vi "Lab Panel V4.82.vi"() -> ()   [LabVIEW 2013] (continued)
                            n1335 = Bundle(cluster=w2277) -> (w2276:T4)  [unwired: 3 in]
                            n1336 = local write "DISP LAB01-1"(w2276) -> ()
                            n1337 = local write "O/I  LAB01-1"(w2274) -> ()
                            n1338 = local write "run lab01-1"(w2274) -> ()
                            n1339 = local write "RUN LAB01-1"(w2274) -> ()
                          }
                          frame #1 {
                            n1340 = TDMS Close(11:w2279) -> (0:w2278:errorcluster)  [unwired: 1 in, 1 out]
                            n1341 = local write "data file error"(w2278) -> ()
                          }
                          frame #2 {
                            n1342 = stacked-sequence {
                              tunnel: "LAB01-1" -> [w2282 w2284]
                              frame #0 {
                                n1343 = call "sub vi - defrag tdms v1.vi"("panel id"=w2282) -> ("error out"=w2281:errorcluster)  [unwired: 10 in]
                                n1344 = local write "data file error"(w2281) -> ()
                              }
                              frame #1 {
                                n1345 = call "Save data file to network drive v1.vi"("panel id"=w2284) -> ("network file save error"=w2283:errorcluster)  [unwired: 9 in, 1 out]
                                n1346 = local write "data file error"(w2283) -> ()
                              }
                            }
                          }
                        }
                      }
                    }
                  }
                }
              }
              frame #1 {
                # "LAB01-2"
                n1347 = local read "run lab01-2"() -> (w2285:bool)
                n1348 = case shown="True" w2285 {
                  frame False {
                  }
                  frame True {
                    n1349 = local read "DISP LAB01-2"() -> (w2292:T4)
                    n1350 = local read "TDMS LAB01-2"() -> (w2291:refnum<k34>)
                    n1351 = Unbundle(w2292) -> ("CYCLE"=w2288:dbl, "STATUS"=w2293:string)  [unwired: 1 out]
                    n1352 = Not Equal?(x=w2293, y="RUN") -> (x != y?=w2287:bool)
                    n1353 = Greater?(x=w2288, y=2.0) -> (0:w2289:bool)
                    n1354 = And(x=w2289, y=w2287) -> (x .and. y?=w2286:bool)
                    n1355 = case shown="True" w2286 {
                      tunnel: w2292 -> [_ w2296]
                      tunnel: w2291 -> [_ w2295]
                      frame False {
                      }
                      frame True {
                        n1356 = stacked-sequence {
                          tunnel: w2296 -> [w2299 _ _]
                          tunnel: w2295 -> [_ w2301 _]
                          frame #0 {
                            w2297 = FALSE
                            n1357 = local write "mail control"("END") -> ()
                            n1358 = Bundle(cluster=w2299) -> (w2300:T4)  [unwired: 3 in]
                            n1359 = local write "RUN LAB01-2"(w2297) -> ()
                            n1360 = local write "run lab01-2"(w2297) -> ()
                            n1361 = local write "O/I  LAB01-2"(w2297) -> ()
                            n1362 = local write "DISP LAB01-2"(w2300) -> ()
                          }
                          frame #1 {
                            n1363 = TDMS Close(11:w2301) -> (0:w2302:errorcluster)  [unwired: 1 in, 1 out]
                            n1364 = local write "data file error"(w2302) -> ()
                          }
                          frame #2 {
                            n1365 = stacked-sequence {
                              tunnel: "LAB01-2" -> [w2305 w2307]
                              frame #0 {
                                n1366 = call "sub vi - defrag tdms v1.vi"("panel id"=w2305) -> ("error out"=w2304:errorcluster)  [unwired: 10 in]
                                n1367 = local write "data file error"(w2304) -> ()
                              }
                              frame #1 {
                                n1368 = call "Save data file to network drive v1.vi"("panel id"=w2307) -> ("network file save error"=w2306:errorcluster)  [unwired: 9 in, 1 out]
                                n1369 = local write "data file error"(w2306) -> ()
                              }
                            }
                          }
                        }
                      }
                    }
                  }
                }
              }
              frame #2 {
                # "LAB02-1"
                n1370 = local read "run lab02-1"() -> (w2308:bool)
                n1371 = case shown="True" w2308 {
                  frame False {
                  }
                  frame True {
                    n1372 = local read "DISP LAB02-1"() -> (w2315:T4)
                    n1373 = Unbundle(w2315) -> ("CYCLE"=w2311:dbl, "STATUS"=w2316:string)  [unwired: 1 out]
                    n1374 = local read "TDMS LAB02-1"() -> (w2314:refnum<k34>)
                    n1375 = Not Equal?(x=w2316, y="RUN") -> (x != y?=w2310:bool)
                    n1376 = Greater?(x=w2311, y=2.0) -> (0:w2312:bool)
                    n1377 = And(x=w2312, y=w2310) -> (x .and. y?=w2309:bool)
                    n1378 = case shown="True" w2309 {
                      tunnel: w2315 -> [_ w2319]
                      tunnel: w2314 -> [_ w2318]
                      frame False {
                      }
                      frame True {
                        n1379 = stacked-sequence {
                          tunnel: w2319 -> [w2322 _ _]
                          tunnel: w2318 -> [_ w2324 _]
                          frame #0 {
                            w2320 = FALSE
                            n1380 = local write "mail control"("END") -> ()
                            n1381 = Bundle(cluster=w2322) -> (w2323:T4)  [unwired: 3 in]
                            n1382 = local write "O/I  LAB02-1"(w2320) -> ()
                            n1383 = local write "RUN LAB02-1"(w2320) -> ()
                            n1384 = local write "run lab02-1"(w2320) -> ()
                            n1385 = local write "DISP LAB02-1"(w2323) -> ()
                          }
                          frame #1 {
                            n1386 = TDMS Close(11:w2324) -> (0:w2325:errorcluster)  [unwired: 1 in, 1 out]
                            n1387 = local write "data file error"(w2325) -> ()
                          }
                          frame #2 {
                            n1388 = stacked-sequence {
                              tunnel: "LAB02-1" -> [w2328 w2330]
                              frame #0 {
                                n1389 = call "sub vi - defrag tdms v1.vi"("panel id"=w2328) -> ("error out"=w2327:errorcluster)  [unwired: 10 in]
                                n1390 = local write "data file error"(w2327) -> ()
                              }
                              frame #1 {
                                n1391 = call "Save data file to network drive v1.vi"("panel id"=w2330) -> ("network file save error"=w2329:errorcluster)  [unwired: 9 in, 1 out]
                                n1392 = local write "data file error"(w2329) -> ()
                              }
                            }
                          }
                        }
                      }
                    }
                  }
                }
              }
              frame #3 {
                # "LAB02-2"
                n1393 = local read "run lab02-2"() -> (w2331:bool)
                n1394 = case shown="True" w2331 {
                  frame False {
                  }
                  frame True {
                    n1395 = local read "DISP LAB02-2"() -> (w2338:T4)
                    n1396 = local read "TDMS LAB02-2"() -> (w2337:refnum<k34>)
                    n1397 = Unbundle(w2338) -> ("CYCLE"=w2334:dbl, "STATUS"=w2339:string)  [unwired: 1 out]
                    n1398 = Not Equal?(x=w2339, y="RUN") -> (x != y?=w2333:bool)
                    n1399 = Greater?(x=w2334, y=2.0) -> (0:w2335:bool)
                    n1400 = And(x=w2335, y=w2333) -> (x .and. y?=w2332:bool)
                    n1401 = case shown="True" w2332 {
                      tunnel: w2338 -> [_ w2342]
                      tunnel: w2337 -> [_ w2341]
                      frame False {
                      }
                      frame True {
                        n1402 = stacked-sequence {
                          tunnel: w2342 -> [w2345 _ _]
                          tunnel: w2341 -> [_ w2347 _]
                          frame #0 {
                            w2343 = FALSE
                            n1403 = local write "mail control"("END") -> ()
                            n1404 = Bundle(cluster=w2345) -> (w2346:T4)  [unwired: 3 in]
                            n1405 = local write "O/I  LAB02-2"(w2343) -> ()
                            n1406 = local write "run lab02-2"(w2343) -> ()
                            n1407 = local write "RUN LAB02-2"(w2343) -> ()
                            n1408 = local write "DISP LAB02-2"(w2346) -> ()
                          }
                          frame #1 {
                            n1409 = TDMS Close(11:w2347) -> (0:w2348:errorcluster)  [unwired: 1 in, 1 out]
                            n1410 = local write "data file error"(w2348) -> ()
                          }
                          frame #2 {
                            n1411 = stacked-sequence {
                              tunnel: "LAB02-2" -> [w2351 w2353]
                              frame #0 {
                                n1412 = call "sub vi - defrag tdms v1.vi"("panel id"=w2351) -> ("error out"=w2350:errorcluster)  [unwired: 10 in]
                                n1413 = local write "data file error"(w2350) -> ()
                              }
                              frame #1 {
                                n1414 = call "Save data file to network drive v1.vi"("panel id"=w2353) -> ("network file save error"=w2352:errorcluster)  [unwired: 9 in, 1 out]
                                n1415 = local write "data file error"(w2352) -> ()
                              }
                            }
                          }
                        }
                      }
                    }
                  }
                }
              }
              frame #4 {
                # "LAB03-1"
                n1416 = local read "run lab03-1"() -> (w2354:bool)
                n1417 = case shown="True" w2354 {
                  frame False {
                  }
                  frame True {
                    n1418 = local read "DISP LAB03-1"() -> (w2361:T4)
                    n1419 = local read "TDMS LAB03-1"() -> (w2360:refnum<k34>)
                    n1420 = Unbundle(w2361) -> ("CYCLE"=w2357:dbl, "STATUS"=w2362:string)  [unwired: 1 out]
                    n1421 = Not Equal?(x=w2362, y="RUN") -> (x != y?=w2356:bool)
                    n1422 = Greater?(x=w2357, y=2.0) -> (0:w2358:bool)
                    n1423 = And(x=w2358, y=w2356) -> (x .and. y?=w2355:bool)
                    n1424 = case shown="True" w2355 {
                      tunnel: w2361 -> [_ w2365]
                      tunnel: w2360 -> [_ w2364]
                      frame False {
                      }
                      frame True {
                        n1425 = stacked-sequence {
                          tunnel: w2365 -> [w2368 _ _]
                          tunnel: w2364 -> [_ w2370 _]
                          frame #0 {
                            w2366 = FALSE
                            n1426 = local write "mail control"("END") -> ()
                            n1427 = Bundle(cluster=w2368) -> (w2369:T4)  [unwired: 3 in]
                            n1428 = local write "O/I  LAB03-1"(w2366) -> ()
                            n1429 = local write "run lab03-1"(w2366) -> ()
                            n1430 = local write "RUN LAB03-1"(w2366) -> ()
                            n1431 = local write "DISP LAB03-1"(w2369) -> ()
                          }
                          frame #1 {
                            n1432 = TDMS Close(11:w2370) -> (0:w2371:errorcluster)  [unwired: 1 in, 1 out]
                            n1433 = local write "data file error"(w2371) -> ()
                          }
                          frame #2 {
                            n1434 = stacked-sequence {
                              tunnel: "LAB03-1" -> [w2374 w2376]
                              frame #0 {
                                n1435 = call "sub vi - defrag tdms v1.vi"("panel id"=w2374) -> ("error out"=w2373:errorcluster)  [unwired: 10 in]
                                n1436 = local write "data file error"(w2373) -> ()
                              }
                              frame #1 {
                                n1437 = call "Save data file to network drive v1.vi"("panel id"=w2376) -> ("network file save error"=w2375:errorcluster)  [unwired: 9 in, 1 out]
                                n1438 = local write "data file error"(w2375) -> ()
                              }
                            }
                          }
                        }
                      }
                    }
                  }
                }
              }
              frame #5 {
                # "LAB03-2"
                n1439 = local read "run lab03-2"() -> (w2377:bool)
                n1440 = case shown="True" w2377 {
                  frame False {
                  }
                  frame True {
                    n1441 = local read "DISP LAB03-2"() -> (w2384:T4)
                    n1442 = Unbundle(w2384) -> ("CYCLE"=w2380:dbl, "STATUS"=w2385:string)  [unwired: 1 out]
                    n1443 = local read "TDMS LAB03-2"() -> (w2383:refnum<k34>)
                    n1444 = Not Equal?(x=w2385, y="RUN") -> (x != y?=w2379:bool)
                    n1445 = Greater?(x=w2380, y=2.0) -> (0:w2381:bool)
                    n1446 = And(x=w2381, y=w2379) -> (x .and. y?=w2378:bool)
                    n1447 = case shown="True" w2378 {
                      tunnel: w2384 -> [_ w2388]
                      tunnel: w2383 -> [_ w2387]
                      frame False {
                      }
                      frame True {
                        n1448 = stacked-sequence {
                          tunnel: w2388 -> [w2391 _ _]
                          tunnel: w2387 -> [_ w2393 _]
                          frame #0 {
                            w2389 = FALSE
                            n1449 = local write "mail control"("END") -> ()
                            n1450 = Bundle(cluster=w2391) -> (w2392:T4)  [unwired: 3 in]
                            n1451 = local write "RUN LAB03-2"(w2389) -> ()
                            n1452 = local write "O/I  LAB03-2"(w2389) -> ()
                            n1453 = local write "DISP LAB03-2"(w2392) -> ()
                            n1454 = local write "run lab03-2"(w2389) -> ()
                          }
                          frame #1 {
                            n1455 = TDMS Close(11:w2393) -> (0:w2394:errorcluster)  [unwired: 1 in, 1 out]
                            n1456 = local write "data file error"(w2394) -> ()
                          }
                          frame #2 {
                            n1457 = stacked-sequence {
                              tunnel: "LAB03-2" -> [w2397 w2399]
                              frame #0 {
                                n1458 = call "sub vi - defrag tdms v1.vi"("panel id"=w2397) -> ("error out"=w2396:errorcluster)  [unwired: 10 in]
                                n1459 = local write "data file error"(w2396) -> ()
                              }
                              frame #1 {
                                n1460 = call "Save data file to network drive v1.vi"("panel id"=w2399) -> ("network file save error"=w2398:errorcluster)  [unwired: 9 in, 1 out]
                                n1461 = local write "data file error"(w2398) -> ()
                              }
                            }
                          }
                        }
                      }
                    }
                  }
                }
              }
              frame #6 {
                # "LAB04-1"
                n1462 = local read "run lab04-1"() -> (w2400:bool)
                n1463 = case shown="True" w2400 {
                  frame False {
                  }
                  frame True {
                    n1464 = local read "DISP LAB04-1"() -> (w2407:T4)
                    n1465 = Unbundle(w2407) -> ("CYCLE"=w2403:dbl, "STATUS"=w2408:string)  [unwired: 1 out]
                    n1466 = local read "TDMS LAB04-1"() -> (w2406:refnum<k34>)
                    n1467 = Not Equal?(x=w2408, y="RUN") -> (x != y?=w2402:bool)
                    n1468 = Greater?(x=w2403, y=2.0) -> (0:w2404:bool)
                    n1469 = And(x=w2404, y=w2402) -> (x .and. y?=w2401:bool)
                    n1470 = case shown="True" w2401 {
                      tunnel: w2407 -> [_ w2411]
                      tunnel: w2406 -> [_ w2410]
                      frame False {
                      }
                      frame True {
                        n1471 = stacked-sequence {
                          tunnel: w2411 -> [w2414 _ _]
                          tunnel: w2410 -> [_ w2416 _]
                          frame #0 {
                            w2412 = FALSE
                            n1472 = local write "mail control"("END") -> ()
                            n1473 = Bundle(cluster=w2414) -> (w2415:T4)  [unwired: 3 in]
                            n1474 = local write "RUN LAB04-1"(w2412) -> ()
                            n1475 = local write "O/I  LAB04-1"(w2412) -> ()
                            n1476 = local write "run lab04-1"(w2412) -> ()
                            n1477 = local write "DISP LAB04-1"(w2415) -> ()
                          }
                          frame #1 {
                            n1478 = TDMS Close(11:w2416) -> (0:w2417:errorcluster)  [unwired: 1 in, 1 out]
                            n1479 = local write "data file error"(w2417) -> ()
                          }
                          frame #2 {
                            n1480 = stacked-sequence {
                              tunnel: "LAB04-1" -> [w2420 w2422]
                              frame #0 {
                                n1481 = call "sub vi - defrag tdms v1.vi"("panel id"=w2420) -> ("error out"=w2419:errorcluster)  [unwired: 10 in]
                                n1482 = local write "data file error"(w2419) -> ()
                              }
                              frame #1 {
                                n1483 = call "Save data file to network drive v1.vi"("panel id"=w2422) -> ("network file save error"=w2421:errorcluster)  [unwired: 9 in, 1 out]
                                n1484 = local write "data file error"(w2421) -> ()
                              }
                            }
                          }
                        }
                      }
                    }
                  }
                }
              }
              frame #7 {
                # "LAB04-2"
                n1485 = local read "run lab04-2"() -> (w2423:bool)
                n1486 = case shown="True" w2423 {
                  frame False {
                  }
                  frame True {
                    n1487 = local read "DISP LAB04-2"() -> (w2430:T4)
                    n1488 = Unbundle(w2430) -> ("CYCLE"=w2426:dbl, "STATUS"=w2431:string)  [unwired: 1 out]
                    n1489 = Not Equal?(x=w2431, y="RUN") -> (x != y?=w2425:bool)
                    n1490 = local read "TDMS LAB04-2"() -> (w2429:refnum<k34>)
                    n1491 = Greater?(x=w2426, y=2.0) -> (0:w2427:bool)
                    n1492 = And(x=w2427, y=w2425) -> (x .and. y?=w2424:bool)
                    n1493 = case shown="True" w2424 {
                      tunnel: w2430 -> [_ w2434]
                      tunnel: w2429 -> [_ w2433]
                      frame False {
                      }
                      frame True {
                        n1494 = stacked-sequence {
                          tunnel: w2434 -> [w2437 _ _]
                          tunnel: w2433 -> [_ w2439 _]
                          frame #0 {
                            w2435 = FALSE
                            n1495 = local write "mail control"("END") -> ()
                            n1496 = Bundle(cluster=w2437) -> (w2438:T4)  [unwired: 3 in]
                            n1497 = local write "O/I  LAB04-2"(w2435) -> ()
                            n1498 = local write "RUN LAB04-2"(w2435) -> ()
                            n1499 = local write "run lab04-2"(w2435) -> ()
                            n1500 = local write "DISP LAB04-2"(w2438) -> ()
                          }
                          frame #1 {
                            n1501 = TDMS Close(11:w2439) -> (0:w2440:errorcluster)  [unwired: 1 in, 1 out]
                            n1502 = local write "data file error"(w2440) -> ()
                          }
                          frame #2 {
                            n1503 = stacked-sequence {
                              tunnel: "LAB04-2" -> [w2443 w2445]
                              frame #0 {
                                n1504 = call "sub vi - defrag tdms v1.vi"("panel id"=w2443) -> ("error out"=w2442:errorcluster)  [unwired: 10 in]
                                n1505 = local write "data file error"(w2442) -> ()
                              }
                              frame #1 {
                                n1506 = call "Save data file to network drive v1.vi"("panel id"=w2445) -> ("network file save error"=w2444:errorcluster)  [unwired: 9 in, 1 out]
                                n1507 = local write "data file error"(w2444) -> ()
                              }
                            }
                          }
                        }
                      }
                    }
                  }
                }
              }
              frame #8 {
                # "LAB05-1"
                n1508 = local read "run lab05-1"() -> (w2446:bool)
                n1509 = case shown="True" w2446 {
                  frame False {
                  }
                  frame True {
                    n1510 = local read "DISP LAB05-1"() -> (w2453:T4)
                    n1511 = Unbundle(w2453) -> ("CYCLE"=w2449:dbl, "STATUS"=w2454:string)  [unwired: 1 out]
                    n1512 = Not Equal?(x=w2454, y="RUN") -> (x != y?=w2448:bool)
                    n1513 = local read "TDMS LAB05-1"() -> (w2452:refnum<k34>)
                    n1514 = Greater?(x=w2449, y=2.0) -> (0:w2450:bool)
                    n1515 = And(x=w2450, y=w2448) -> (x .and. y?=w2447:bool)
                    n1516 = case shown="True" w2447 {
                      tunnel: w2453 -> [_ w2457]
                      tunnel: w2452 -> [_ w2456]
                      frame False {
                      }
                      frame True {
                        n1517 = stacked-sequence {
                          tunnel: w2457 -> [w2460 _ _]
                          tunnel: w2456 -> [_ w2462 _]
                          frame #0 {
                            w2458 = FALSE
                            n1518 = local write "mail control"("END") -> ()
                            n1519 = Bundle(cluster=w2460) -> (w2461:T4)  [unwired: 3 in]
                            n1520 = local write "O/I  LAB05-1"(w2458) -> ()
                            n1521 = local write "RUN LAB05-1"(w2458) -> ()
                            n1522 = local write "run lab05-1"(w2458) -> ()
                            n1523 = local write "DISP LAB05-1"(w2461) -> ()
                          }
                          frame #1 {
                            n1524 = TDMS Close(11:w2462) -> (0:w2463:errorcluster)  [unwired: 1 in, 1 out]
                            n1525 = local write "data file error"(w2463) -> ()
                          }
                          frame #2 {
                            n1526 = stacked-sequence {
                              tunnel: "LAB05-1" -> [w2466 w2468]
                              frame #0 {
                                n1527 = call "sub vi - defrag tdms v1.vi"("panel id"=w2466) -> ("error out"=w2465:errorcluster)  [unwired: 10 in]
                                n1528 = local write "data file error"(w2465) -> ()
                              }
                              frame #1 {
                                n1529 = call "Save data file to network drive v1.vi"("panel id"=w2468) -> ("network file save error"=w2467:errorcluster)  [unwired: 9 in, 1 out]
                                n1530 = local write "data file error"(w2467) -> ()
                              }
                            }
                          }
                        }
                      }
                    }
                  }
                }
              }
              frame #9 {
                # "LAB05-2"
                n1531 = local read "run lab05-2"() -> (w2469:bool)
                n1532 = case shown="True" w2469 {
                  frame False {
                  }
                  frame True {
                    n1533 = local read "DISP LAB05-2"() -> (w2476:T4)
                    n1534 = Unbundle(w2476) -> ("CYCLE"=w2472:dbl, "STATUS"=w2477:string)  [unwired: 1 out]
                    n1535 = Not Equal?(x=w2477, y="RUN") -> (x != y?=w2471:bool)
                    n1536 = local read "TDMS LAB05-2"() -> (w2475:refnum<k34>)
                    n1537 = Greater?(x=w2472, y=2.0) -> (0:w2473:bool)
                    n1538 = And(x=w2473, y=w2471) -> (x .and. y?=w2470:bool)
                    n1539 = case shown="True" w2470 {
                      tunnel: w2476 -> [_ w2480]
                      tunnel: w2475 -> [_ w2479]
                      frame False {
                      }
                      frame True {
                        n1540 = stacked-sequence {
                          tunnel: w2480 -> [w2483 _ _]
                          tunnel: w2479 -> [_ w2485 _]
                          frame #0 {
                            w2481 = FALSE
                            n1541 = local write "mail control"("END") -> ()
                            n1542 = Bundle(cluster=w2483) -> (w2484:T4)  [unwired: 3 in]
                            n1543 = local write "RUN LAB05-2"(w2481) -> ()
                            n1544 = local write "O/I  LAB05-2"(w2481) -> ()
                            n1545 = local write "run lab05-2"(w2481) -> ()
                            n1546 = local write "DISP LAB05-2"(w2484) -> ()
                          }
                          frame #1 {
                            n1547 = TDMS Close(11:w2485) -> (0:w2486:errorcluster)  [unwired: 1 in, 1 out]
                            n1548 = local write "data file error"(w2486) -> ()
                          }
                          frame #2 {
                            n1549 = stacked-sequence {
                              tunnel: "LAB05-2" -> [w2489 w2491]
                              frame #0 {
                                n1550 = call "sub vi - defrag tdms v1.vi"("panel id"=w2489) -> ("error out"=w2488:errorcluster)  [unwired: 10 in]
                                n1551 = local write "data file error"(w2488) -> ()
                              }
                              frame #1 {
                                n1552 = call "Save data file to network drive v1.vi"("panel id"=w2491) -> ("network file save error"=w2490:errorcluster)  [unwired: 9 in, 1 out]
                                n1553 = local write "data file error"(w2490) -> ()
                              }
                            }
                          }
                        }
                      }
                    }
                  }
                }
              }
            }
            n1554 = local read "Network Directory"() -> (w2247:path)
            n1555 = global write "Global 1.vi" "Network Drive"(w2247) -> ()
          }
          frame #7 {
            # "disable functions"
            n1556 = stacked-sequence {
              tunnel: w2501 -> [w2515 _ w2571]
              tunnel: w2500 -> [w2510 _ w2570]
              tunnel: w2499 -> [w2509 _ w2569]
              tunnel: w2498 -> [w2507 _ w2568]
              tunnel: w2497 -> [w2508 _ w2567]
              tunnel: w2496 -> [_ w2532 w2566]
              tunnel: w2495 -> [_ w2533 w2565]
              tunnel: w2494 -> [_ w2534 w2564]
              tunnel: w2493 -> [_ w2535 w2563]
              tunnel: w2492 -> [_ w2536 w2562]
              frame #0 {
                n1557 = Select(t=2, s=w2507, f=0) -> (s? t:f=w2503:i32)
                n1558 = Select(t=2, s=w2509, f=0) -> (s? t:f=w2504:i32)
                n1559 = Select(t=2, s=w2508, f=0) -> (s? t:f=w2502:i32)
                n1560 = Select(t=2, s=w2515, f=0) -> (s? t:f=w2506:i32)
                n1561 = Select(t=2, s=w2510, f=0) -> (s? t:f=w2505:i32)
                n1562 = property on="SELECT LAB02-2" class="RadioBtnsControl (strict)"("DisabledEnum"=w2503) -> ()  [unwired: 2 in, 2 out]
                n1563 = property on="SELECT LAB02-1" class="RadioBtnsControl (strict)"("DisabledEnum"=w2504) -> ()  [unwired: 2 in, 2 out]
                n1564 = property on="SELECT LAB03-1" class="RadioBtnsControl (strict)"("DisabledEnum"=w2502) -> ()  [unwired: 2 in, 2 out]
                n1565 = property on="SELECT LAB01-1" class="RadioBtnsControl (strict)"("DisabledEnum"=w2506) -> ()  [unwired: 2 in, 2 out]
                n1566 = property on="SELECT LAB01-2" class="RadioBtnsControl (strict)"("DisabledEnum"=w2505) -> ()  [unwired: 2 in, 2 out]
                n1567 = Not(x=w2515) -> (.not. x?=w2516:bool)
                n1568 = property on="RESULT LAB01-1" class="Bool (strict)"("Visible"=w2516) -> ()  [unwired: 2 in, 2 out]
                n1569 = Not(x=w2510) -> (.not. x?=w2514:bool)
                n1570 = Not(x=w2509) -> (.not. x?=w2513:bool)
                n1571 = Not(x=w2507) -> (.not. x?=w2512:bool)
                n1572 = property on="RESULT LAB01-2" class="Bool (strict)"("Visible"=w2514) -> ()  [unwired: 2 in, 2 out]
                n1573 = Not(x=w2508) -> (.not. x?=w2511:bool)
                n1574 = property on="RESULT LAB02-1" class="Bool (strict)"("Visible"=w2513) -> ()  [unwired: 2 in, 2 out]
                n1575 = property on="RESULT LAB02-2" class="Bool (strict)"("Visible"=w2512) -> ()  [unwired: 2 in, 2 out]
                n1576 = property on="RESULT LAB03-1" class="Bool (strict)"("Visible"=w2511) -> ()  [unwired: 2 in, 2 out]
                n1577 = property on="SET LAB01-1" class="Clust (strict)"("DisabledEnum"=w2506) -> ()  [unwired: 2 in, 2 out]
                n1578 = property on="SET LAB01-2" class="Clust (strict)"("DisabledEnum"=w2505) -> ()  [unwired: 2 in, 2 out]
                n1579 = property on="SET LAB02-1" class="Clust (strict)"("DisabledEnum"=w2504) -> ()  [unwired: 2 in, 2 out]
                n1580 = property on="SET LAB02-2" class="Clust (strict)"("DisabledEnum"=w2503) -> ()  [unwired: 2 in, 2 out]
                n1581 = property on="SET LAB03-1" class="Clust (strict)"("DisabledEnum"=w2502) -> ()  [unwired: 2 in, 2 out]
                n1582 = property on="O/I  LAB01-1" class="Bool (strict)"("DisabledEnum"=w2506) -> ()  [unwired: 2 in, 2 out]
                n1583 = property on="O/I  LAB01-2" class="Bool (strict)"("DisabledEnum"=w2505) -> ()  [unwired: 2 in, 2 out]
                n1584 = property on="O/I  LAB02-1" class="Bool (strict)"("DisabledEnum"=w2504) -> ()  [unwired: 2 in, 2 out]
                n1585 = property on="O/I  LAB02-2" class="Bool (strict)"("DisabledEnum"=w2503) -> ()  [unwired: 2 in, 2 out]
                n1586 = property on="O/I  LAB03-1" class="Bool (strict)"("DisabledEnum"=w2502) -> ()  [unwired: 2 in, 2 out]
              }
              frame #1 {
                n1587 = Select(t=2, s=w2536, f=0) -> (s? t:f=w2527:i32)
                n1588 = Select(t=2, s=w2535, f=0) -> (s? t:f=w2528:i32)
                n1589 = Select(t=2, s=w2532, f=0) -> (s? t:f=w2531:i32)
                n1590 = Select(t=2, s=w2533, f=0) -> (s? t:f=w2530:i32)
                n1591 = Select(t=2, s=w2534, f=0) -> (s? t:f=w2529:i32)
                n1592 = property on="SELECT LAB05-2" class="RadioBtnsControl (strict)"("DisabledEnum"=w2527) -> ()  [unwired: 2 in, 2 out]
                n1593 = property on="SELECT LAB05-1" class="RadioBtnsControl (strict)"("DisabledEnum"=w2528) -> ()  [unwired: 2 in, 2 out]
                n1594 = property on="SELECT LAB03-2" class="RadioBtnsControl (strict)"("DisabledEnum"=w2531) -> ()  [unwired: 2 in, 2 out]
                n1595 = property on="SELECT LAB04-1" class="RadioBtnsControl (strict)"("DisabledEnum"=w2530) -> ()  [unwired: 2 in, 2 out]
                n1596 = property on="SELECT LAB04-2" class="RadioBtnsControl (strict)"("DisabledEnum"=w2529) -> ()  [unwired: 2 in, 2 out]
                n1597 = property on="SET LAB05-2" class="Clust (strict)"("DisabledEnum"=w2527) -> ()  [unwired: 2 in, 2 out]
                n1598 = property on="SET LAB05-1" class="Clust (strict)"("DisabledEnum"=w2528) -> ()  [unwired: 2 in, 2 out]
                n1599 = property on="SET LAB03-2" class="Clust (strict)"("DisabledEnum"=w2531) -> ()  [unwired: 2 in, 2 out]
                n1600 = property on="SET LAB04-1" class="Clust (strict)"("DisabledEnum"=w2530) -> ()  [unwired: 2 in, 2 out]
                n1601 = property on="SET LAB04-2" class="Clust (strict)"("DisabledEnum"=w2529) -> ()  [unwired: 2 in, 2 out]
                n1602 = property on="O/I  LAB05-2" class="Bool (strict)"("DisabledEnum"=w2527) -> ()  [unwired: 2 in, 2 out]
                n1603 = property on="O/I  LAB05-1" class="Bool (strict)"("DisabledEnum"=w2528) -> ()  [unwired: 2 in, 2 out]
                n1604 = property on="O/I  LAB04-1" class="Bool (strict)"("DisabledEnum"=w2530) -> ()  [unwired: 2 in, 2 out]
                n1605 = property on="O/I  LAB04-2" class="Bool (strict)"("DisabledEnum"=w2529) -> ()  [unwired: 2 in, 2 out]
                n1606 = property on="O/I  LAB03-2" class="Bool (strict)"("DisabledEnum"=w2531) -> ()  [unwired: 2 in, 2 out]
                n1607 = Not(x=w2536) -> (.not. x?=w2537:bool)
                n1608 = Not(x=w2535) -> (.not. x?=w2538:bool)
                n1609 = Not(x=w2534) -> (.not. x?=w2539:bool)
                n1610 = property on="RESULT LAB05-2" class="Bool (strict)"("Visible"=w2537) -> ()  [unwired: 2 in, 2 out]
                n1611 = property on="RESULT LAB05-1" class="Bool (strict)"("Visible"=w2538) -> ()  [unwired: 2 in, 2 out]
                n1612 = Not(x=w2533) -> (.not. x?=w2540:bool)
                n1613 = property on="RESULT LAB04-2" class="Bool (strict)"("Visible"=w2539) -> ()  [unwired: 2 in, 2 out]
                n1614 = Not(x=w2532) -> (.not. x?=w2541:bool)
                n1615 = property on="RESULT LAB04-1" class="Bool (strict)"("Visible"=w2540) -> ()  [unwired: 2 in, 2 out]
                n1616 = property on="RESULT LAB03-2" class="Bool (strict)"("Visible"=w2541) -> ()  [unwired: 2 in, 2 out]
              }
              frame #2 {
                # "disable calibrate if any test running"
                n1617 = Or(x=w2563, y=w2562) -> (x .or. y?=w2556:bool)
                n1618 = Or(x=w2565, y=w2564) -> (x .or. y?=w2558:bool)
                n1619 = Or(x=w2569, y=w2568) -> (x .or. y?=w2560:bool)
                n1620 = Or(x=w2567, y=w2566) -> (x .or. y?=w2559:bool)
                n1621 = Or(x=w2571, y=w2570) -> (x .or. y?=w2561:bool)
                n1622 = Or(x=w2559, y=w2558) -> (x .or. y?=w2557:bool)
                n1623 = Or(x=w2561, y=w2560) -> (x .or. y?=w2555:bool)
                n1624 = Or(x=w2557, y=w2556) -> (x .or. y?=w2554:bool)
                n1625 = Or(x=w2555, y=w2554) -> (x .or. y?=w2553:bool)
                n1626 = case shown="True" w2553 {
                  tunnel: [0 2] -> w2552
                  frame False {
                  }
                  frame True {
                  }
                }
                n1627 = property on="JIG TEST" class="Clust (strict)"("DisabledEnum"=w2552) -> ()  [unwired: 2 in, 2 out]
                n1628 = property on="Network Directory" class="Path"("DisabledEnum"=w2552) -> ()  [unwired: 2 in, 2 out]
                n1629 = property on="MAIL SETTINGS" class="Clust (strict)"("DisabledEnum"=w2552) -> ()  [unwired: 2 in, 2 out]
                n1630 = property on="CALIBRATE" class="Bool (strict)"("DisabledEnum"=w2552) -> ()  [unwired: 2 in, 2 out]
                n1631 = property on="ADMIN PAGE" class="Bool (strict)"("DisabledEnum"=w2552) -> ()  [unwired: 2 in, 2 out]
              }
            }
          }
          frame #8 {
            # "drive jigs"
            n1632 = stacked-sequence {
              frame #0 {
                # "jig on"
                n1633 = local read "jig cycle"() -> (w2579:dbl)
                n1634 = property on="JIG TEST" class="Clust (strict)"() -> ("DisabledEnum"=w2576:T15)  [unwired: 2 in, 2 out]
                n1635 = Equal?(x=w2576, y=2) -> (x = y?=w2575:bool)
                n1636 = Equal?(x=w2579, y=0) -> (x = y?=w2577:bool)
                n1637 = And(x=w2577, y=w2575) -> (x .and. y?=w2574:bool)
                n1638 = case shown="True" w2574 {
                  frame False {
                  }
                  frame True {
                    n1639 = local read "run lab01-1"() -> (w2590:bool)
                    n1640 = local read "run lab01-2"() -> (w2589:bool)
                    n1641 = local read "run lab02-1"() -> (w2588:bool)
                    n1642 = local read "run lab02-2"() -> (w2587:bool)
                    n1643 = local read "run lab03-1"() -> (w2586:bool)
                    n1644 = local read "run lab03-2"() -> (w2585:bool)
                    n1645 = local read "run lab04-1"() -> (w2584:bool)
                    n1646 = local read "run lab04-2"() -> (w2583:bool)
                    n1647 = local read "run lab05-1"() -> (w2582:bool)
                    n1648 = local read "run lab05-2"() -> (w2581:bool)
                    n1649 = local write "JIG LAB03-2"(w2585) -> ()
                    n1650 = local write "JIG LAB01-1"(w2590) -> ()
                    n1651 = local write "JIG LAB01-2"(w2589) -> ()
                    n1652 = local write "JIG LAB02-1"(w2588) -> ()
                    n1653 = local write "JIG LAB02-2"(w2587) -> ()
                    n1654 = local write "JIG LAB03-1"(w2586) -> ()
                    n1655 = local write "JIG LAB04-1"(w2584) -> ()
                    n1656 = local write "JIG LAB04-2"(w2583) -> ()
                    n1657 = local write "JIG LAB05-1"(w2582) -> ()
                    n1658 = local write "JIG LAB05-2"(w2581) -> ()
                  }
                }
              }
              frame #1 {
                # "jig off"
                n1659 = local read "jig cycle"() -> (w2597:dbl)
                n1660 = local read "on loops"() -> (w2596:dbl)
                n1661 = property on="JIG TEST" class="Clust (strict)"() -> ("DisabledEnum"=w2595:T15)  [unwired: 2 in, 2 out]
                n1662 = Equal?(x=w2595, y=2) -> (x = y?=w2593:bool)
                n1663 = Equal?(x=w2597, y=w2596) -> (x = y?=w2592:bool)
                n1664 = And(x=w2592, y=w2593) -> (x .and. y?=w2591:bool)
                n1665 = case shown="True" w2591 {
                  frame False {
                  }
                  frame True {
                    w2648 = FALSE
                    w2649 = TRUE
                    w2647 = 2
                    n1666 = local read "SELECT LAB05-2"() -> (w2638:T3)
                    n1667 = local read "SELECT LAB04-2"() -> (w2640:T3)
                    n1668 = local read "SELECT LAB04-1"() -> (w2641:T3)
                    n1669 = local read "SELECT LAB05-1"() -> (w2639:T3)
                    n1670 = local read "SELECT LAB03-2"() -> (w2642:T3)
                    n1671 = local read "SELECT LAB02-1"() -> (w2645:T3)
                    n1672 = local read "SELECT LAB03-1"() -> (w2643:T3)
                    n1673 = local read "SELECT LAB02-2"() -> (w2644:T3)
                    n1674 = local read "SELECT LAB01-2"() -> (w2646:T3)
                    n1675 = local read "run lab05-1"() -> (w2608:bool)
                    n1676 = local read "run lab05-2"() -> (w2607:bool)
                    n1677 = local read "SELECT LAB01-1"() -> (w2650:T3)
                    n1678 = local read "run lab04-2"() -> (w2609:bool)
                    n1679 = local read "run lab04-1"() -> (w2610:bool)
                    n1680 = local read "run lab01-1"() -> (w2626:bool)
                    n1681 = local read "run lab01-2"() -> (w2615:bool)
                    n1682 = local read "run lab03-2"() -> (w2611:bool)
                    n1683 = local read "run lab03-1"() -> (w2612:bool)
                    n1684 = local read "run lab02-1"() -> (w2614:bool)
                    n1685 = local read "run lab02-2"() -> (w2613:bool)
                    n1686 = Equal?(x=w2647, y=w2643) -> (x = y?=w2621:bool)
                    n1687 = Equal?(x=w2647, y=w2642) -> (x = y?=w2620:bool)
                    n1688 = Equal?(x=w2647, y=w2641) -> (x = y?=w2619:bool)
                    n1689 = Equal?(x=w2647, y=w2640) -> (x = y?=w2618:bool)
                    n1690 = Equal?(x=w2647, y=w2639) -> (x = y?=w2617:bool)
                    n1691 = Equal?(x=w2647, y=w2638) -> (x = y?=w2616:bool)
                    n1692 = Equal?(x=w2647, y=w2650) -> (x = y?=w2627:bool)
                    n1693 = Equal?(x=w2647, y=w2645) -> (x = y?=w2623:bool)
                    n1694 = Equal?(x=w2647, y=w2644) -> (x = y?=w2622:bool)
                    n1695 = Equal?(x=w2647, y=w2646) -> (x = y?=w2624:bool)
                    n1696 = And(x=w2618, y=w2609) -> (x .and. y?=w2600:bool)
                    n1697 = And(x=w2621, y=w2612) -> (x .and. y?=w2603:bool)
                    n1698 = And(x=w2619, y=w2610) -> (x .and. y?=w2601:bool)
                    n1699 = And(x=w2616, y=w2607) -> (x .and. y?=w2598:bool)
                    n1700 = And(x=w2622, y=w2613) -> (x .and. y?=w2604:bool)
                    n1701 = And(x=w2620, y=w2611) -> (x .and. y?=w2602:bool)
                    n1702 = And(x=w2617, y=w2608) -> (x .and. y?=w2599:bool)
                    n1703 = And(x=w2624, y=w2615) -> (x .and. y?=w2606:bool)
                    n1704 = And(x=w2627, y=w2626) -> (x .and. y?=w2625:bool)
                    n1705 = And(x=w2623, y=w2614) -> (x .and. y?=w2605:bool)
                    n1706 = Select(t=w2649, s=w2625, f=w2648) -> (s? t:f=w2628:bool)
                    n1707 = Select(t=w2649, s=w2606, f=w2648) -> (s? t:f=w2629:bool)
                    n1708 = Select(t=w2649, s=w2605, f=w2648) -> (s? t:f=w2630:bool)
                    n1709 = Select(t=w2649, s=w2604, f=w2648) -> (s? t:f=w2631:bool)
                    n1710 = Select(t=w2649, s=w2603, f=w2648) -> (s? t:f=w2632:bool)
                    n1711 = Select(t=w2649, s=w2602, f=w2648) -> (s? t:f=w2633:bool)
                    n1712 = Select(t=w2649, s=w2601, f=w2648) -> (s? t:f=w2634:bool)
                    n1713 = Select(t=w2649, s=w2600, f=w2648) -> (s? t:f=w2635:bool)
                    n1714 = Select(t=w2649, s=w2599, f=w2648) -> (s? t:f=w2636:bool)
                    n1715 = Select(t=w2649, s=w2598, f=w2648) -> (s? t:f=w2637:bool)
                    n1716 = local write "JIG LAB03-2"(w2633) -> ()
                    n1717 = local write "JIG LAB02-1"(w2630) -> ()
                    n1718 = local write "JIG LAB02-2"(w2631) -> ()
                    n1719 = local write "JIG LAB01-2"(w2629) -> ()
                    n1720 = local write "JIG LAB03-1"(w2632) -> ()
                    n1721 = local write "JIG LAB01-1"(w2628) -> ()
                    n1722 = local write "JIG LAB05-2"(w2637) -> ()
                    n1723 = local write "JIG LAB04-1"(w2634) -> ()
                    n1724 = local write "JIG LAB05-1"(w2636) -> ()
                    n1725 = local write "JIG LAB04-2"(w2635) -> ()
                  }
                }
              }
            }
          }
          frame #9 {
            # "enable  jig test output if no test busy"
            n1726 = property on="JIG TEST" class="Clust (strict)"() -> ("DisabledEnum"=w2653:T15)  [unwired: 2 in, 2 out]
            n1727 = Equal?(x=w2653, y=0) -> (x = y?=w2651:bool)
            n1728 = case shown="True" w2651 {
              frame False {
              }
              frame True {
                n1729 = local read "JIG TEST"() -> (w2664:T12)
                n1730 = Unbundle(w2664) -> ("LAB01-1"=w2663:bool, "LAB01-2"=w2662:bool, "LAB02-1"=w2661:bool, "LAB02-2"=w2660:bool, "LAB03-1"=w2659:bool, "LAB03-2"=w2658:bool, "LAB04-1"=w2657:bool, "LAB04-2"=w2656:bool, "LAB05-1"=w2655:bool, "LAB05-2"=w2654:bool)
                n1731 = local write "JIG LAB05-1"(w2655) -> ()
                n1732 = local write "JIG LAB05-2"(w2654) -> ()
                n1733 = local write "JIG LAB04-1"(w2657) -> ()
                n1734 = local write "JIG LAB04-2"(w2656) -> ()
                n1735 = local write "JIG LAB03-2"(w2658) -> ()
                n1736 = local write "JIG LAB01-1"(w2663) -> ()
                n1737 = local write "JIG LAB02-1"(w2661) -> ()
                n1738 = local write "JIG LAB03-1"(w2659) -> ()
                n1739 = local write "JIG LAB01-2"(w2662) -> ()
                n1740 = local write "JIG LAB02-2"(w2660) -> ()
              }
            }
          }
          frame #10 {
            # "drive digital output"
            n1741 = local read "O/I  LAB05-2"() -> (w2671:bool)
            n1742 = local read "O/I  LAB05-1"() -> (w2673:bool)
            n1743 = local read "JIG LAB05-2"() -> (w2670:bool)
            n1744 = local read "O/I  LAB04-2"() -> (w2675:bool)
            n1745 = local read "JIG LAB05-1"() -> (w2672:bool)
            n1746 = local read "JIG LAB04-2"() -> (w2674:bool)
            n1747 = local read "O/I  LAB03-1"() -> (w2680:bool)
            n1748 = local read "O/I  LAB04-1"() -> (w2676:bool)
            n1749 = local read "O/I  LAB02-1"() -> (w2684:bool)
            n1750 = local read "O/I  LAB02-2"() -> (w2682:bool)
            n1751 = local read "O/I  LAB03-2"() -> (w2678:bool)
            n1752 = local read "JIG LAB04-1"() -> (w2669:bool)
            n1753 = local read "JIG LAB03-2"() -> (w2677:bool)
            n1754 = local read "O/I  LAB01-2"() -> (w2686:bool)
            n1755 = local read "JIG LAB02-1"() -> (w2683:bool)
            n1756 = local read "JIG LAB02-2"() -> (w2681:bool)
            n1757 = local read "JIG LAB03-1"() -> (w2679:bool)
            n1758 = local read "O/I  LAB01-1"() -> (w2688:bool)
            n1759 = local read "JIG LAB01-2"() -> (w2685:bool)
            n1760 = local read "JIG LAB01-1"() -> (w2687:bool)
            n1761 = Build Array(w2675, w2674, w2673, w2672, w2671, w2670) -> (w2666:bool[])
            n1762 = Build Array(w2681, w2680, w2679, w2678, w2677, w2676, w2669) -> (w2667:bool[])
            n1763 = Build Array(w2688, w2687, w2686, w2685, w2684, w2683, w2682) -> (w2668:bool[])
            n1764 = local read "simulate"() -> (w2665:bool)
            n1765 = case shown="False" w2665 {
              tunnel: w2668 -> [w2691 _]
              tunnel: w2667 -> [w2690 _]
              tunnel: w2666 -> [w2689 _]
              frame False {
                n1766 = call "sub vi - Drive Relays All v6.vi"("Array #2"=w2689, "Array #1"=w2690, "Array #0"=w2691) -> ()  [unwired: 8 in, 1 out]
              }
              frame True {
              }
            }
          }
          frame #11 {
            # "get analog values"
            n1767 = local read "on loops"() -> (w2698:dbl)
            n1768 = local read "jig cycle"() -> (w2695:dbl)
            n1769 = Add(x=w2698, y=1) -> (x+y=w2696:dbl)
            n1770 = Equal?(x=w2695, y=1) -> (x = y?=w2693:bool)
            n1771 = Equal?(x=w2695, y=w2696) -> (x = y?=w2694:bool)
            n1772 = Or(x=w2693, y=w2694) -> (x .or. y?=w2692:bool)
            n1773 = case shown="True" w2692 {
              frame False {
              }
              frame True {
                n1774 = local read "simulate"() -> (w2702:bool)
                n1775 = case shown="False" w2702 {
                  tunnel: [w2718 errorcluster[] [] ("array ERROR")] -> w2710
                  tunnel: [w2717 0.3 ("Analog loop time")] -> w2709
                  tunnel: [w2716 dynamicdata[] [] ("array GRAPH")] -> w2708
                  tunnel: [w2715 w2720] -> w2707
                  tunnel: [w2714 w2720] -> w2706
                  tunnel: [w2713 w2720] -> w2705
                  tunnel: [w2712 w2720] -> w2704
                  tunnel: [w2711 w2720] -> w2703
                  frame False {
                    n1776 = call "sub vi - Read Analog All v8.vi"() -> ("Analog loop time"=w2717:dbl, "array GRAPH"=w2716:dynamicdata[], "LAB01"=w2715:T24, "LAB02"=w2714:T25, "LAB03"=w2713:T26, "LAB04"=w2712:T27, "array ERROR"=w2718:errorcluster[], "LAB05"=w2711:T28)  [unwired: 8 in]
                  }
                  frame True {
                    w2720 = T28 {"LAB05-1 (A)"=10.0, "LAB05-1 (V)"=220.0, "LAB05-1 (PF)"=0.5, "LAB05-2 (A)"=15.0, "LAB05-2 (V)"=225.0, "LAB05-2 (PF)"=0.6} ("LAB05")
                  }
                }
                n1777 = local read "simulate"() -> (w2701:bool)
                n1778 = stacked-sequence {
                  tunnel: w2710 -> [w2727 _ _ _ _ _]
                  tunnel: w2709 -> [w2726 _ _ _ _ _]
                  tunnel: w2708 -> [w2725 _ _ _ _ _]
                  tunnel: w2707 -> [_ w2774 _ _ _ _]
                  tunnel: w2706 -> [_ _ w2779 _ _ _]
                  tunnel: w2705 -> [_ _ _ w2808 _ _]
                  tunnel: w2704 -> [_ _ _ _ w2835 _]
                  tunnel: w2703 -> [_ _ _ _ _ w2864]
                  tunnel: w2701 -> [_ w2750 w2778 w2806 w2834 w2862]
                  tunnel: T8 {"1  (A) cal"=1.0, "1 (V) cal"=1.0, "1 (PF) cal"=1.0, "1 (TL) cal"=1.0, "1 (TN) cal"=1.0, "2 (A) cal"=1.0, "2 (V) cal"=1.0, "2 (PF) cal"=1.0, "2 (TL) cal"=1.0, "2 (TN) cal"=1.0} ("CAL LAB01") -> [_ w2749 w2777 w2805 w2833 w2861]
                  frame #0 {
                    n1779 = local write "AI update"(TRUE) -> ()
